vi "Build home command.vi"(8 "error in (no error)":errorcluster, 10 "Home direction (M2)":T1 items=["", "Forward", "Backward"], 11 "Home direction (M1)":T1 items=["", "Forward", "Backward"]) -> (0 "error out":errorcluster, 3 "String":string)   [LabVIEW 2020, in "Arduino-Adafruit stepper.lvlib"]
uses:
  Arduino-Adafruit stepper.lvlib
  Arduino stepper library/Public/Controls/Motor direction.ctl
  Arduino stepper library/Control de MaP.lvlib
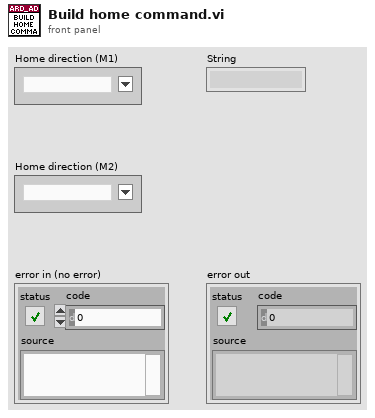
[diagram p1: front panel]
types:
  T1 = typedef "Control de MaP.lvlib/Motor direction.ctl" = u8
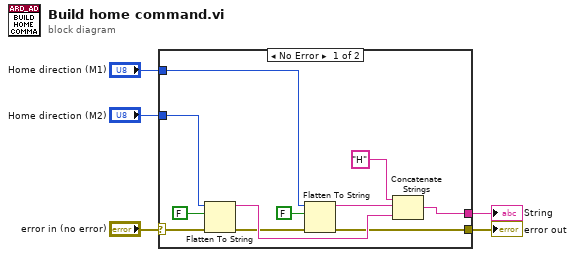
[diagram p0: block diagram]
diagram:
  n1 = case shown="No Error" "error in (no error)" {
    selector: "error in (no error)" -> [w16 w17]
    tunnel: "Home direction (M2)" -> [w14 _]
    tunnel: [w11 _] -> w3
    tunnel: "Home direction (M1)" -> [w8 _]
    tunnel: [w7 w17] -> w1
    frame No Error {
      n2 = Flatten To String(anything=w14, prepend array or string size? (T)=FALSE, error in (no error)=w16) -> (data string=w15:string, error out=w13:errorcluster)  [unwired: 1 in, 1 out]
      n3 = Flatten To String(anything=w8, prepend array or string size? (T)=FALSE, error in (no error)=w13) -> (data string=w9:string, error out=w7:errorcluster)  [unwired: 1 in, 1 out]
      n4 = Concatenate Strings("H", w9, w15) -> (w11:string)
    }
    frame Error {
    }
  }
  "String" <- w3
  "error out" <- w1
